vi "http create status string.vi"(10 "status string":string, 11 "reason code":u16) -> (3 "status line":string)   [LabVIEW 2013, in "http headers.lvlib"]
uses:
  http headers.lvlib
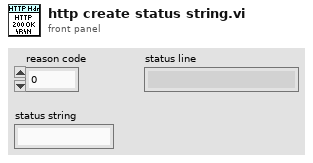
[diagram p1: front panel]
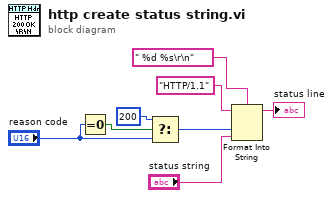
[diagram p0: block diagram]
diagram:
  n1 = Equal To 0?(x="reason code") -> (x = 0?=w5:bool)
  n2 = Select(t=u16 200, s=w5, f="reason code") -> (s? t:f=w1:u16)
  n3 = Format Into String(format string=" %d %s\r\n", initial string="HTTP/1.1" ("input 1"), w1, "status string") -> (resulting string=→"status line":string)  [unwired: 1 in, 1 out]
